vi "Tree Value Change.vi"(10 "Selection Changed?":bool, 11 "UI Data in":refnum<class "Settings UI.lvclass">) -> (3 "UI Data out":refnum<class "Settings UI.lvclass">)   [LabVIEW 2020, in "Output Sequencer.lvlib" / "Settings UI.lvclass"]
uses:
  Settings UI.lvclass
  Settings UI.lvclass/Settings UI.ctl
  <vilib>/Utility/miscctls.llb/LVPositionTypeDef.ctl
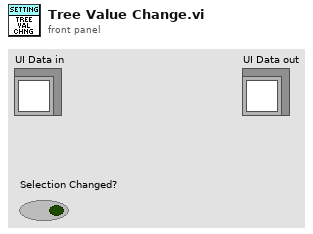
[diagram p1: front panel]
types:
  T1 = typedef "Output Sequencer.lvlib/Settings UI.lvclass/Data Type.ctl" = i16
  T2 = typedef "LVPositionTypeDef.ctl" = cluster{"Left":i32, "Top":i32}
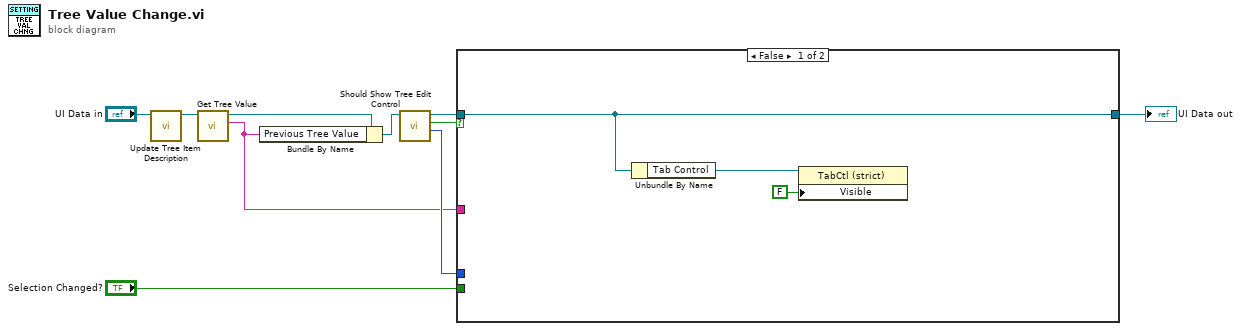
[diagram p0: block diagram]
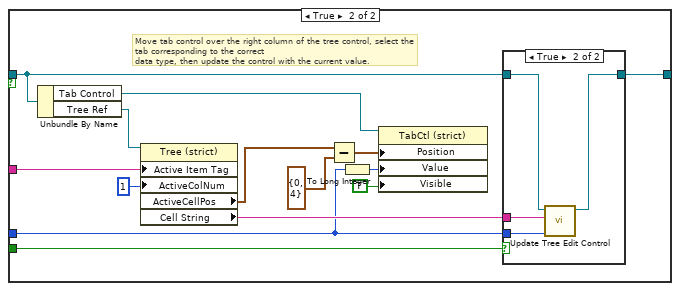
[diagram p2: hidden frame]
diagram:
  n1 = call "Update Tree Item Description.vi"("UI Data in"="UI Data in") -> ("UI Data out"=w3:refnum<class "Settings UI.lvclass">)  [unwired: 10 in]
  n2 = call "Get Tree Value.vi"("UI Data in"=w3) -> ("Value"=w6:string, "UI Data out"=w2:refnum<class "Settings UI.lvclass">)  [unwired: 9 in]
  n3 = Bundle By Name(cluster=w2, "Previous Tree Value"=w6) -> (w1:refnum<class "Settings UI.lvclass">)
  n4 = call "Should Show Tree Edit Control.vi"("UI Data in"=w1) -> ("Data Type"=w8:T1, "Show Tree Edit Control"=w9:bool, "UI Data out"=w4:refnum<class "Settings UI.lvclass">)  [unwired: 8 in]
  n5 = case shown="False" w9 {
    tunnel: w8 -> [_ w14]
    tunnel: w4 -> [w11 w16]
    tunnel: "Selection Changed?" -> [_ w23]
    tunnel: w6 -> [_ w22]
    tunnel: [w11 w15] -> w5
    frame False {
      n6 = Unbundle By Name(w11) -> ("Tab Control"=w12:refnum<vi>)
      n7 = property class="TabCtl (strict)"(reference=w12, "Visible"=FALSE) -> ()  [unwired: 1 in, 2 out]
    }
    frame True {
      # "Move tab control over the right column of the tree control, select the tab corresponding to the correct\ndata type, then update the control with the current value."
      n8 = Unbundle By Name(w16) -> ("Tab Control"=w18:refnum<vi>, "Tree Ref"=w17:refnum<vi>)
      n9 = property class="Tree (strict)"(reference=w17, "Active Item Tag"=w22, "ActiveColNum"=1 ("Active Cell:Active Column Number")) -> ("ActiveCellPos"=w20:T2, "Cell String"=w19:string)  [unwired: 1 in, 2 out]
      n10 = Subtract(x=w20, y=T2 {"Left"=0, "Top"=4}) -> (x-y=w25:T2)
      n11 = To Long Integer(number=w14) -> (32bit integer=w27:i32)
      n12 = property class="TabCtl (strict)"(reference=w18, "Position"=w25, "Value"=w27, "Visible"=TRUE) -> ()  [unwired: 1 in, 2 out]
      n13 = case shown="True" w23 {
        tunnel: w16 -> [w28 w32]
        tunnel: w19 -> [_ w31]
        tunnel: [w28 w30] -> w15
        tunnel: w14 -> [_ w29]
        frame False {
        }
        frame True {
          n14 = call "Update Tree Edit Control.vi"("Data Type"=w29, "Value"=w31, "UI Data in"=w32) -> ("UI Data out"=w30:refnum<class "Settings UI.lvclass">)  [unwired: 8 in]
        }
      }
    }
  }
  "UI Data out" <- w5
